vi "JoinRects.vi"(1 "Rect in 2":T1, 2 "Rect in 1":T1) -> (0 "Rect out":T1)   [LabVIEW 2016]
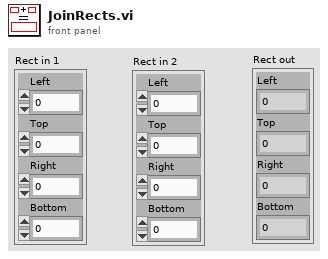
[diagram p1: front panel]
types:
  T1 = cluster{"Left":dbl, "Top":dbl, "Right":dbl, "Bottom":dbl}
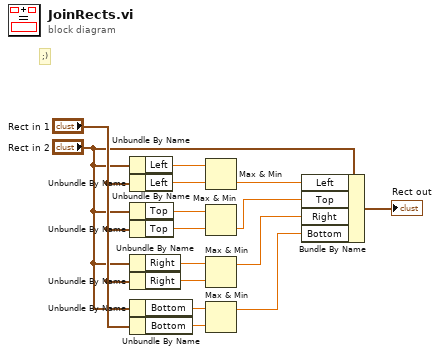
[diagram p0: block diagram]
diagram:
  # ";)"
  n1 = Unbundle By Name("Rect in 2") -> ("Left"=w15:dbl)
  n2 = Unbundle By Name("Rect in 1") -> ("Left"=w14:dbl)
  n3 = Unbundle By Name("Rect in 2") -> ("Top"=w12:dbl)
  n4 = Unbundle By Name("Rect in 1") -> ("Top"=w11:dbl)
  n5 = Unbundle By Name("Rect in 2") -> ("Right"=w9:dbl)
  n6 = Unbundle By Name("Rect in 1") -> ("Right"=w8:dbl)
  n7 = Unbundle By Name("Rect in 2") -> ("Bottom"=w6:dbl)
  n8 = Unbundle By Name("Rect in 1") -> ("Bottom"=w5:dbl)
  n9 = Max & Min(x=w15, y=w14) -> (min(x,y)=w13:dbl)  [unwired: 1 out]
  n10 = Max & Min(x=w12, y=w11) -> (min(x,y)=w10:dbl)  [unwired: 1 out]
  n11 = Max & Min(x=w9, y=w8) -> (max(x,y)=w7:dbl)  [unwired: 1 out]
  n12 = Max & Min(x=w6, y=w5) -> (max(x,y)=w3:dbl)  [unwired: 1 out]
  n13 = Bundle By Name(cluster="Rect in 2", "Left"=w13, "Top"=w10, "Right"=w7, "Bottom"=w3) -> (→"Rect out":T1)
